vi "SUB-ROM Data convert to table.vi"(4 "ROM Table Ref":refnum<vi>, 5 "ROM Data Ref":refnum<vi>) -> (1 "ROM Table":string[][](table)=[["Device ID", "-", "-"], ["Main Chip", "-", "-"], ["YEAR", "-", "-"], ["Month", "-", "-"], ["Day", "-", "-"], ["Device Type", "-", "-"], ["Manufacturer ID", "-", "-"], ["Cal_Acc. X", "-", "-"], ["Cal_Acc. Y", "-", "-"], ["Cal_Acc. Z", "-", "-"], ["Cal_Gy. X", "-", "-"], ["Cal_Gy. Y", "-", "-"], ["Cal_Gy. Z", "-", "-"], ["Cal_Vol H", "-", "-"], ["Cal_Vol L", "-", "-"], ["Cal_CDC Off 1", "-", "-"], ["Cal_CDC Off 2", "-", "-"], ["Cal_CDC Off 3", "-", "-"], ["Cal_CDC Off 4", "-", "-"], ["Cal_CDC Off 5", "-", "-"], ["Cal_CDC Off 6", "-", "-"], ["Cal_CDC Gain A", "-", "-"], ["Cal_CDC Gain B", "-", "-"]], 2 "ROM Data":T1(array[cluster])=[{"RxOK"=TRUE, "ROM Data"=[255, 255, 255, 255, 255, 255, 255, 255, 255, 255, 255, 255, 255, 255, 255, 255, 2], "Index"=0}, {"RxOK"=TRUE, "ROM Data"=[255, 255, 255, 255, 255, 255, 255, 255, 255, 255, 255, 255, 255, 255, 255, 255, 5], "Index"=1}, {"RxOK"=TRUE, "ROM Data"=[255, 255, 255, 255, 255, 255, 255, 255, 255, 255, 255, 255, 255, 255, 255, 255, 8], "Index"=2}] {"Index" format="%02x"; "ROM Data" format="%02x"})   [LabVIEW 2015]
panel:
  out "Last Index":i32=2
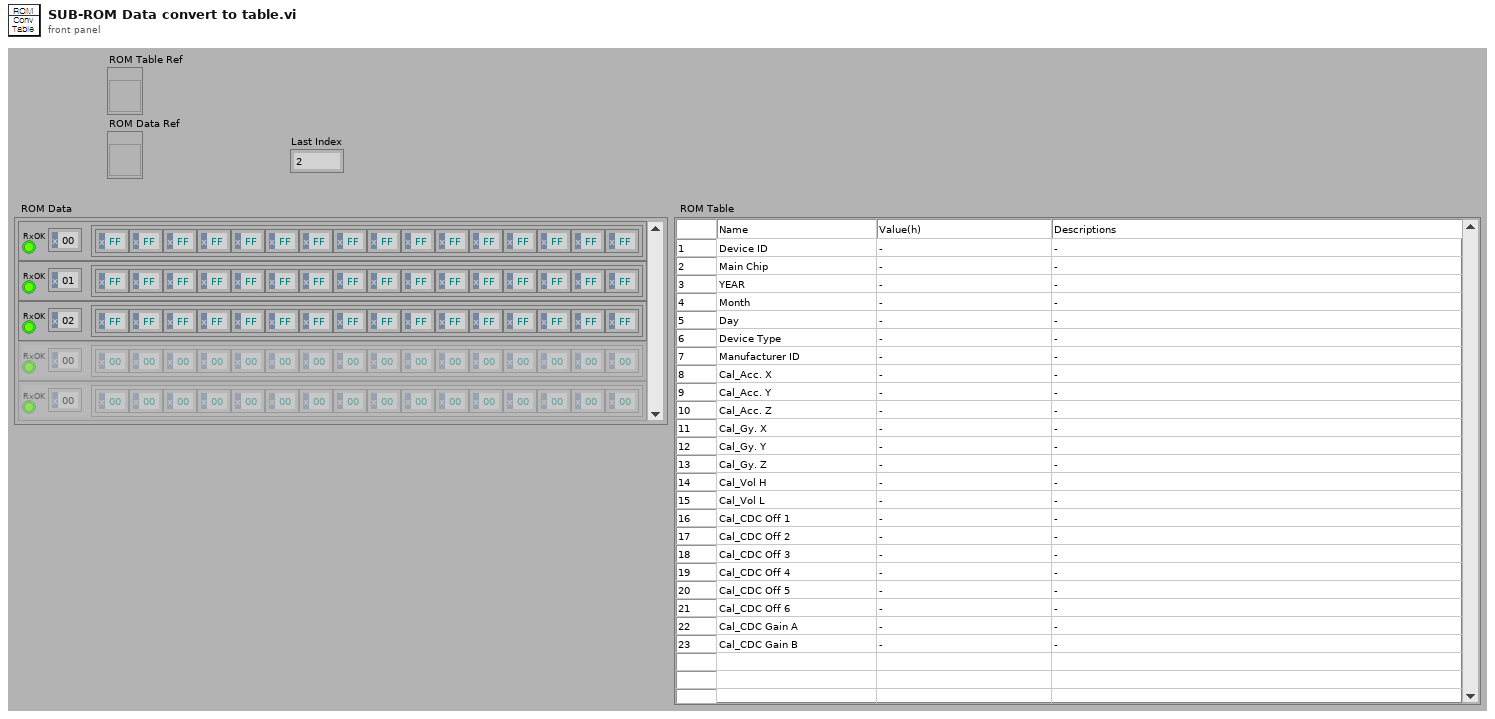
[diagram p1: front panel]
types:
  T1 = cluster{"RxOK":bool, "ROM Data":u8[], "Index":u8}[]
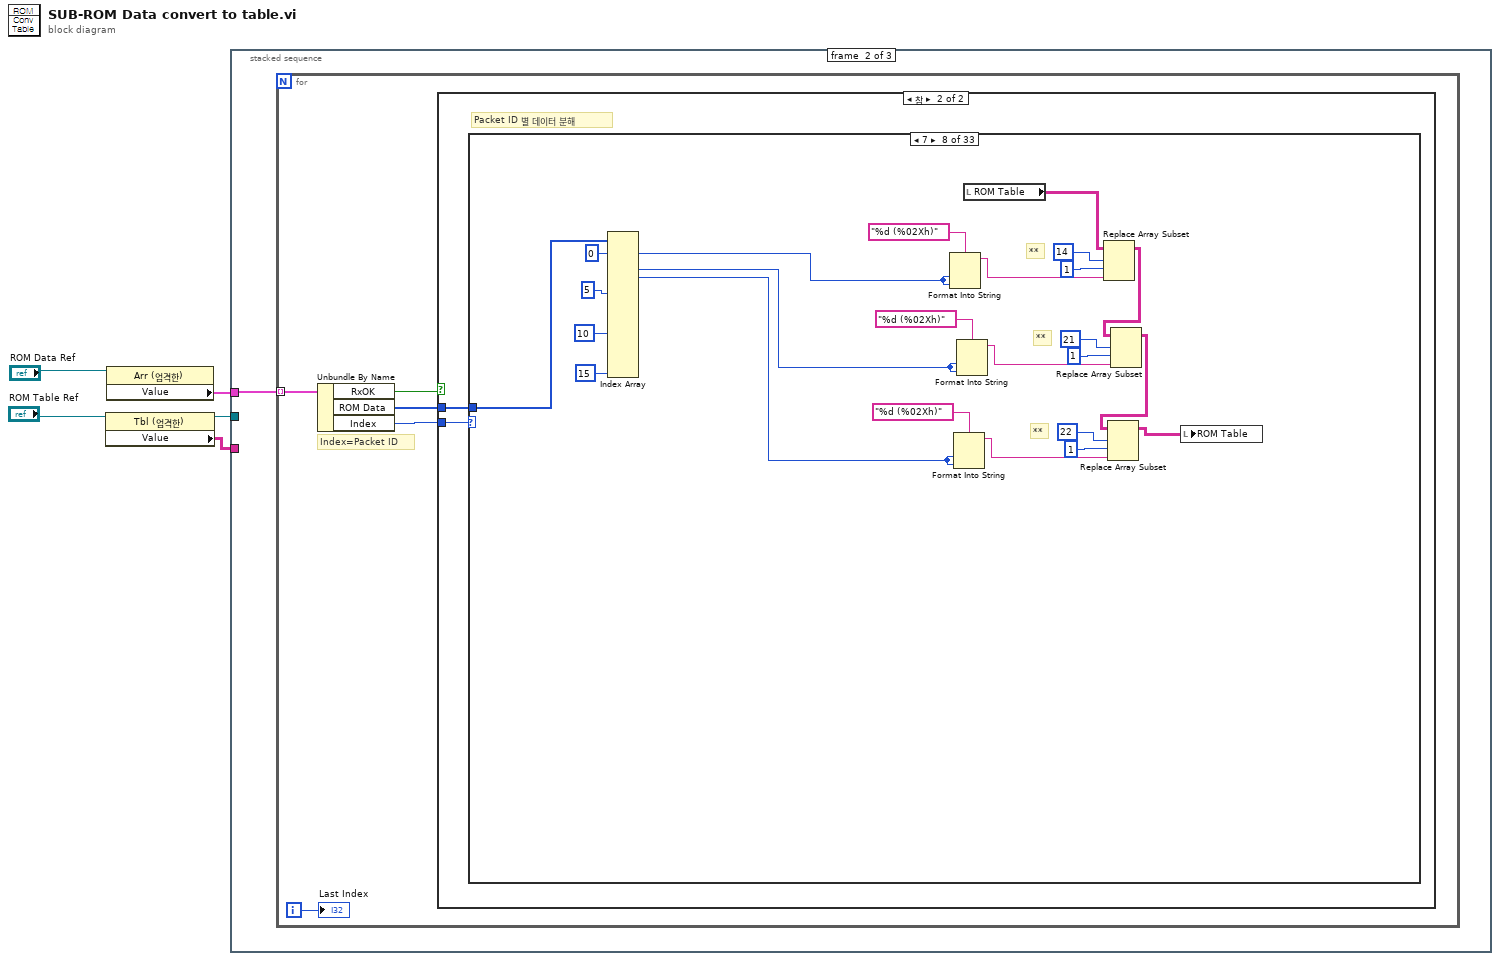
[diagram p0: block diagram]
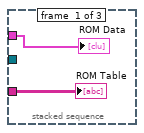
[diagram p2: hidden frame]
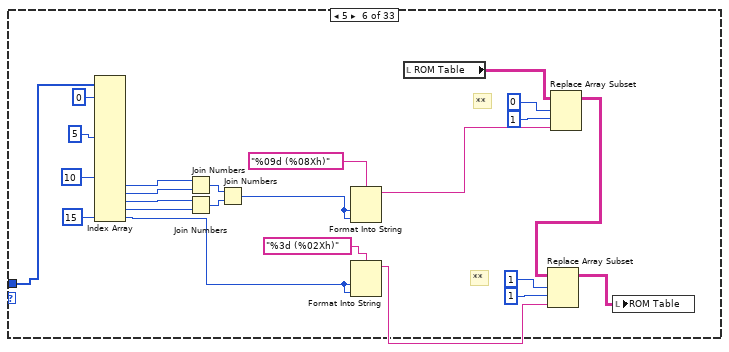
[diagram p9: hidden frame]
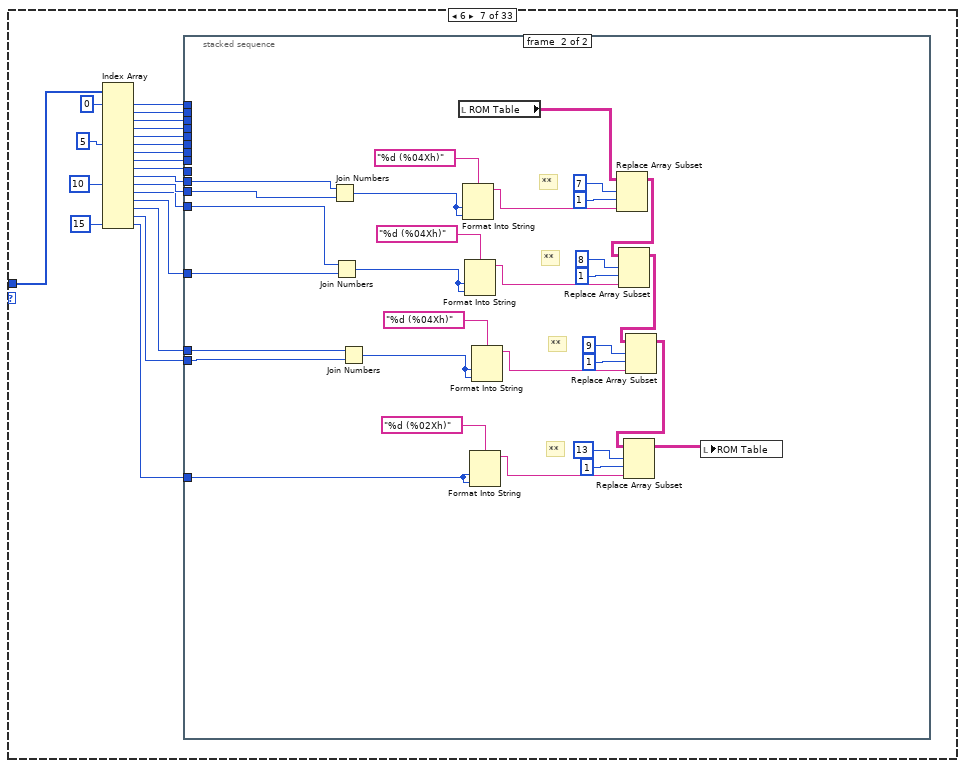
[diagram p10: hidden frame]
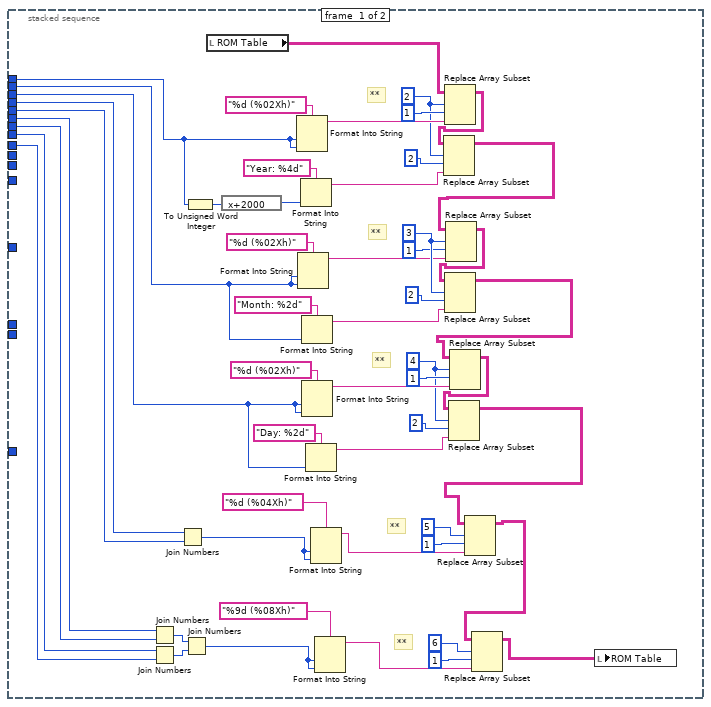
[diagram p11: hidden frame]
diagram:
  n1 = property class="Tbl (엄격한)"(reference="ROM Table Ref") -> (reference out=w1:refnum<vi>, "Value"=w2:string[][])  [unwired: 1 in, 1 out]
  n2 = property class="Arr (엄격한)"(reference="ROM Data Ref") -> ("Value"=w3:T1)  [unwired: 1 in, 2 out]
  n3 = stacked-sequence {
    tunnel: w3 -> [w7 w8 _]
    tunnel: w2 -> [w6 _ _]
    tunnel: w1 -> [_ _ w170]
    frame #0 {
      "ROM Data" <- w7
      "ROM Table" <- w6
    }
    frame #1 {
      n4 = for {
        tunnel: w8 -> [w13] mode=indexing
        i -> [w9]
        # "Index=Packet ID"
        n5 = Unbundle By Name(w13) -> ("RxOK"=w11:bool, "ROM Data"=w10:u8[], "Index"=w12:u8)
        n6 = case shown="참" w11 {
          tunnel: w12 -> [_ w15]
          tunnel: w10 -> [_ w14]
          frame False {
          }
          frame True {
            # "Packet ID 별 데이터 분해"
            n7 = case shown="7" w15 {
              tunnel: w14 -> [_ _ _ _ _ w39 w56 w164 _ _ _ _ _ _ _ _ _ _ _ _ _ _ _ _ _ _ _ _ _ _ _ _ _]
              frame 0 {
              }
              frame 1 {
              }
              frame 2 {
              }
              frame 3 {
              }
              frame 4 {
              }
              frame 5 {
                # "**"
                # "**"
                n8 = Index Array(array=w39, index #1=0 ("인덱스"), index #6=5 ("인덱스"), index #11=10 ("인덱스"), index #16=15 ("인덱스")) -> (element #12=w31:u8, element #13=w30:u8, element #14=w29:u8, element #15=w28:u8, element #16=w17:u8)  [unwired: 12 in, 11 out]
                n9 = Join Numbers(hi=w31, lo=w30) -> ((hi.lo)=w27:u16)
                n10 = Join Numbers(hi=w29, lo=w28) -> ((hi.lo)=w26:u16)
                n11 = Join Numbers(hi=w27, lo=w26) -> ((hi.lo)=w23:u32)
                n12 = Format Into String(format string="%09d (%08Xh)" ("포맷 문자열"), w23, w23) -> (resulting string=w24:string)  [unwired: 2 in, 1 out]
                n13 = Format Into String(format string="%3d (%02Xh)" ("포맷 문자열"), w17, w17) -> (resulting string=w18:string)  [unwired: 2 in, 1 out]
                n14 = local read "ROM Table"() -> (w34:string[][])
                n15 = Replace Array Subset(array=w34, new element=w24, index (row)=0 ("인덱스 (행)"), index (col)=1 ("인덱스 (행)")) -> (w20:string[][])
                n16 = Replace Array Subset(array=w20, new element=w18, index (row)=1 ("인덱스 (행)"), index (col)=1 ("인덱스 (행)")) -> (w19:string[][])
                n17 = local write "ROM Table"(w19) -> ()
              }
              frame 6 {
                n18 = Index Array(array=w56, index #1=0 ("인덱스"), index #6=5 ("인덱스"), index #11=10 ("인덱스"), index #16=15 ("인덱스")) -> (element #1=w55:u8, element #2=w54:u8, element #3=w53:u8, element #4=w52:u8, element #5=w51:u8, element #6=w50:u8, element #7=w49:u8, element #8=w48:u8, element #9=w47:u8, element #10=w46:u8, element #11=w45:u8, element #12=w44:u8, element #13=w43:u8, element #14=w42:u8, element #15=w41:u8, element #16=w40:u8)  [unwired: 12 in]
                n19 = stacked-sequence {
                  tunnel: w55 -> [w102 _]
                  tunnel: w54 -> [w92 _]
                  tunnel: w53 -> [w83 _]
                  tunnel: w52 -> [w75 _]
                  tunnel: w51 -> [w74 _]
                  tunnel: w50 -> [w64 _]
                  tunnel: w49 -> [w63 _]
                  tunnel: w48 -> [w62 _]
                  tunnel: w47 -> [w61 _]
                  tunnel: w46 -> [_ w138]
                  tunnel: w45 -> [_ w137]
                  tunnel: w44 -> [_ w122]
                  tunnel: w43 -> [_ w121]
                  tunnel: w42 -> [_ w120]
                  tunnel: w41 -> [_ w119]
                  tunnel: w40 -> [_ w118]
                  frame #0 {
                    w86 = 4 ("인덱스 (행)")
                    w99 = 3 ("인덱스 (행)")
                    w107 = 2 ("인덱스 (행)")
                    # "**"
                    # "**"
                    # "**"
                    # "**"
                    # "**"
                    n20 = Join Numbers(hi=w64, lo=w63) -> ((hi.lo)=w76:u16)
                    n21 = Join Numbers(hi=w62, lo=w61) -> ((hi.lo)=w77:u16)
                    n22 = Join Numbers(hi=w75, lo=w74) -> ((hi.lo)=w80:u16)
                    n23 = Join Numbers(hi=w76, lo=w77) -> ((hi.lo)=w79:u32)
                    n24 = To Unsigned Word Integer(number=w102) -> (unsigned 16bit integer=w103:u16)
                    n25 = local read "ROM Table"() -> (w113:string[][])
                    n26 = expression code="x+2000"(w103) -> (w104:u16)
                    n27 = Format Into String(format string="%d (%02Xh)" ("포맷 문자열"), w102, w102) -> (resulting string=w110:string)  [unwired: 2 in, 1 out]
                    n28 = Format Into String(format string="%d (%02Xh)" ("포맷 문자열"), w92, w92) -> (resulting string=w96:string)  [unwired: 2 in, 1 out]
                    n29 = Format Into String(format string="Year: %4d" ("포맷 문자열"), w104) -> (resulting string=w105:string)  [unwired: 2 in, 1 out]
                    n30 = Format Into String(format string="Month: %2d" ("포맷 문자열"), w92) -> (resulting string=w101:string)  [unwired: 2 in, 1 out]
                    n31 = Format Into String(format string="%d (%02Xh)" ("포맷 문자열"), w83, w83) -> (resulting string=w89:string)  [unwired: 2 in, 1 out]
                    n32 = Format Into String(format string="Day: %2d" ("포맷 문자열"), w83) -> (resulting string=w84:string)  [unwired: 2 in, 1 out]
                    n33 = Format Into String(format string="%d (%04Xh)" ("포맷 문자열"), w80, w80) -> (resulting string=w70:string)  [unwired: 2 in, 1 out]
                    n34 = Format Into String(format string="%9d (%08Xh)" ("포맷 문자열"), w79, w79) -> (resulting string=w65:string)  [unwired: 2 in, 1 out]
                    n35 = Replace Array Subset(array=w113, new element=w110, index (row)=w107, index (col)=1 ("인덱스 (행)")) -> (w108:string[][])
                    n36 = Replace Array Subset(array=w108, new element=w105, index (row)=w107, index (col)=2 ("인덱스 (행)")) -> (w93:string[][])
                    n37 = Replace Array Subset(array=w93, new element=w96, index (row)=w99, index (col)=1 ("인덱스 (행)")) -> (w98:string[][])
                    n38 = Replace Array Subset(array=w98, new element=w101, index (row)=w99, index (col)=2 ("인덱스 (행)")) -> (w82:string[][])
                    n39 = Replace Array Subset(array=w82, new element=w89, index (row)=w86, index (col)=1 ("인덱스 (행)")) -> (w87:string[][])
                    n40 = Replace Array Subset(array=w87, new element=w84, index (row)=w86, index (col)=2 ("인덱스 (행)")) -> (w71:string[][])
                    n41 = Replace Array Subset(array=w71, new element=w70, index (row)=5 ("인덱스 (행)"), index (col)=1 ("인덱스 (행)")) -> (w67:string[][])
                    n42 = Replace Array Subset(array=w67, new element=w65, index (row)=6 ("인덱스 (행)"), index (col)=1 ("인덱스 (행)")) -> (w66:string[][])
                    n43 = local write "ROM Table"(w66) -> ()
                  }
                  frame #1 {
                    # "**"
                    # "**"
                    # "**"
                    # "**"
                    n44 = Join Numbers(hi=w138, lo=w137) -> ((hi.lo)=w143:u16)
                    n45 = Join Numbers(hi=w122, lo=w121) -> ((hi.lo)=w133:u16)
                    n46 = Join Numbers(hi=w120, lo=w119) -> ((hi.lo)=w130:u16)
                    n47 = local read "ROM Table"() -> (w139:string[][])
                    n48 = Format Into String(format string="%d (%04Xh)" ("포맷 문자열"), w143, w143) -> (resulting string=w140:string)  [unwired: 2 in, 1 out]
                    n49 = Format Into String(format string="%d (%04Xh)" ("포맷 문자열"), w133, w133) -> (resulting string=w136:string)  [unwired: 2 in, 1 out]
                    n50 = Format Into String(format string="%d (%02Xh)" ("포맷 문자열"), w118, w118) -> (resulting string=w126:string)  [unwired: 2 in, 1 out]
                    n51 = Format Into String(format string="%d (%04Xh)" ("포맷 문자열"), w130, w130) -> (resulting string=w127:string)  [unwired: 2 in, 1 out]
                    n52 = Replace Array Subset(array=w139, new element=w140, index (row)=7 ("인덱스 (행)"), index (col)=1 ("인덱스 (행)")) -> (w117:string[][])
                    n53 = Replace Array Subset(array=w117, new element=w136, index (row)=8 ("인덱스 (행)"), index (col)=1 ("인덱스 (행)")) -> (w116:string[][])
                    n54 = Replace Array Subset(array=w116, new element=w127, index (row)=9 ("인덱스 (행)"), index (col)=1 ("인덱스 (행)")) -> (w115:string[][])
                    n55 = Replace Array Subset(array=w115, new element=w126, index (row)=13 ("인덱스 (행)"), index (col)=1 ("인덱스 (행)")) -> (w114:string[][])
                    n56 = local write "ROM Table"(w114) -> ()
                  }
                }
              }
              frame 7 {
                # "**"
                # "**"
                # "**"
                n57 = Index Array(array=w164, index #1=0 ("인덱스"), index #6=5 ("인덱스"), index #11=10 ("인덱스"), index #16=15 ("인덱스")) -> (element #1=w158:u8, element #3=w146:u8, element #4=w145:u8)  [unwired: 12 in, 13 out]
                n58 = Format Into String(format string="%d (%02Xh)" ("포맷 문자열"), w158, w158) -> (resulting string=w162:string)  [unwired: 2 in, 1 out]
                n59 = Format Into String(format string="%d (%02Xh)" ("포맷 문자열"), w145, w145) -> (resulting string=w153:string)  [unwired: 2 in, 1 out]
                n60 = Format Into String(format string="%d (%02Xh)" ("포맷 문자열"), w146, w146) -> (resulting string=w154:string)  [unwired: 2 in, 1 out]
                n61 = local read "ROM Table"() -> (w163:string[][])
                n62 = Replace Array Subset(array=w163, new element=w162, index (row)=14 ("인덱스 (행)"), index (col)=1 ("인덱스 (행)")) -> (w147:string[][])
                n63 = Replace Array Subset(array=w147, new element=w154, index (row)=21 ("인덱스 (행)"), index (col)=1 ("인덱스 (행)")) -> (w148:string[][])
                n64 = Replace Array Subset(array=w148, new element=w153, index (row)=22 ("인덱스 (행)"), index (col)=1 ("인덱스 (행)")) -> (w149:string[][])
                n65 = local write "ROM Table"(w149) -> ()
              }
              frame 8 {
              }
              frame 9 {
              }
              frame 10 {
              }
              frame 11 {
              }
              frame 12 {
              }
              frame 13 {
              }
              frame 14 {
              }
              frame 15 {
              }
              frame 16 {
              }
              frame 17 {
              }
              frame 18 {
              }
              frame 19 {
              }
              frame 20 {
              }
              frame 21 {
              }
              frame 22 {
              }
              frame 23 {
              }
              frame 24 {
              }
              frame 25 {
              }
              frame 26 {
              }
              frame 27 {
              }
              frame 28 {
              }
              frame 29 {
              }
              frame 30 {
              }
              frame 31 {
              }
              frame 100, Default {
              }
            }
          }
        }
        "Last Index" <- w9
      }
    }
    frame #2 {
      n66 = local read "ROM Table"() -> (w169:string[][])
      n67 = property class="Tbl (엄격한)"(reference=w170, "Value"=w169) -> ()  [unwired: 1 in, 2 out]
    }
  }
